vi "Filter and Data Scaling.vi"(5 "Slope":dbl[](array[numeric]), 7 "Offset":dbl[](array[numeric]), 9 "Vin":dbl[](array[numeric]), 11 "error in":errorcluster) -> (4 "Vout":dbl[](array[numeric]), 10 "ScaledOut":dbl[](array[numeric]), 15 "error out":errorcluster)   [LabVIEW 2018]
uses:
  <vilib>/ptbypt/NI_PtbyPt.lvlib
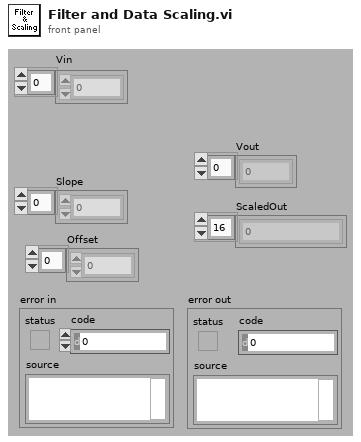
[diagram p1: front panel]
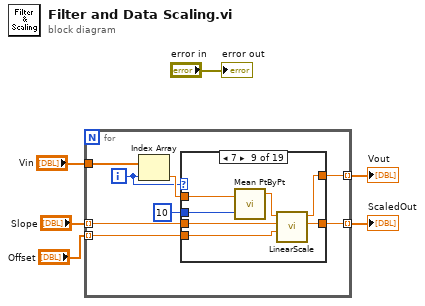
[diagram p0: block diagram]
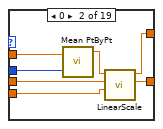
[diagram p3: hidden frame]
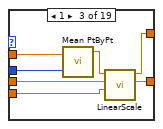
[diagram p4: hidden frame]
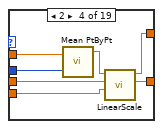
[diagram p5: hidden frame]
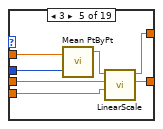
[diagram p6: hidden frame]
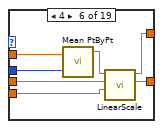
[diagram p7: hidden frame]
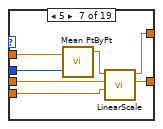
[diagram p8: hidden frame]
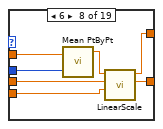
[diagram p9: hidden frame]
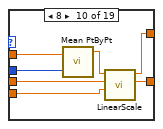
[diagram p10: hidden frame]
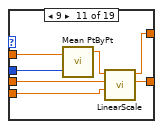
[diagram p11: hidden frame]
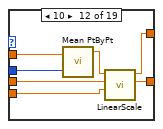
[diagram p12: hidden frame]
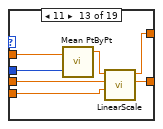
[diagram p13: hidden frame]
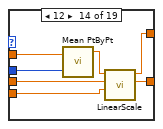
[diagram p14: hidden frame]
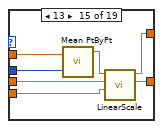
[diagram p15: hidden frame]
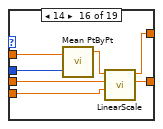
[diagram p16: hidden frame]
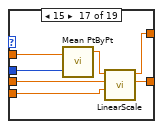
[diagram p17: hidden frame]
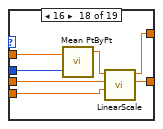
[diagram p18: hidden frame]
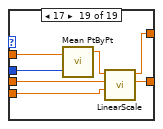
[diagram p19: hidden frame]
diagram:
  n1 = for {
    tunnel: "Slope" -> [w14] mode=indexing
    tunnel: "Offset" -> [w11] mode=indexing
    tunnel: [w12] -> w5 mode=indexing
    tunnel: [w13] -> w1 mode=indexing
    tunnel: "Vin" -> [w10]
    i -> [w8]
    n2 = Index Array(array=w10, index=w8) -> (element=w9:dbl)
    n3 = case shown="7" w8 {
      tunnel: w9 -> [_ w20 w28 w35 w42 w49 w56 w63 w70 w77 w84 w91 w98 w105 w112 w119 w126 w133 w140]
      tunnel: 10 ("String") -> [_ w15 w22 w29 w36 w43 w50 w57 w64 w71 w78 w85 w92 w99 w106 w113 w120 w127 w134]
      tunnel: w14 -> [_ w19 w26 w32 w40 w46 w53 w60 w65 w76 w82 w88 w95 w102 w110 w116 w123 w130 w137]
      tunnel: w11 -> [_ w18 w25 w33 w39 w47 w54 w61 w66 w75 w81 w89 w96 w103 w109 w117 w124 w131 w138]
      tunnel: [_ w16 w23 w31 w38 w45 w52 w59 w68 w73 w80 w87 w94 w101 w108 w115 w122 w129 w136] -> w13
      tunnel: [_ w17 w24 w30 w37 w44 w51 w58 w67 w72 w79 w86 w93 w100 w107 w114 w121 w128 w135] -> w12
      frame Default {
      }
      frame 0 {
        n4 = call <vilib>:"Mean PtByPt.vi"("x"=w20, "sample length"=w15) -> ("mean"=w21:dbl)  [unwired: 1 in, 2 out]
        n5 = call "LinearScale.vi"("Offset"=w18, "Slope"=w19, "Voltage"=w21) -> ("ScaledOut"=w17:dbl, "Vout"=w16:dbl)  [unwired: 7 in]
      }
      frame 1 {
        n6 = call <vilib>:"Mean PtByPt.vi"("x"=w28, "sample length"=w22) -> ("mean"=w27:dbl)  [unwired: 1 in, 2 out]
        n7 = call "LinearScale.vi"("Offset"=w25, "Slope"=w26, "Voltage"=w27) -> ("ScaledOut"=w24:dbl, "Vout"=w23:dbl)  [unwired: 7 in]
      }
      frame 2 {
        n8 = call <vilib>:"Mean PtByPt.vi"("x"=w35, "sample length"=w29) -> ("mean"=w34:dbl)  [unwired: 1 in, 2 out]
        n9 = call "LinearScale.vi"("Offset"=w33, "Slope"=w32, "Voltage"=w34) -> ("ScaledOut"=w30:dbl, "Vout"=w31:dbl)  [unwired: 7 in]
      }
      frame 3 {
        n10 = call <vilib>:"Mean PtByPt.vi"("x"=w42, "sample length"=w36) -> ("mean"=w41:dbl)  [unwired: 1 in, 2 out]
        n11 = call "LinearScale.vi"("Offset"=w39, "Slope"=w40, "Voltage"=w41) -> ("ScaledOut"=w37:dbl, "Vout"=w38:dbl)  [unwired: 7 in]
      }
      frame 4 {
        n12 = call <vilib>:"Mean PtByPt.vi"("x"=w49, "sample length"=w43) -> ("mean"=w48:dbl)  [unwired: 1 in, 2 out]
        n13 = call "LinearScale.vi"("Offset"=w47, "Slope"=w46, "Voltage"=w48) -> ("ScaledOut"=w44:dbl, "Vout"=w45:dbl)  [unwired: 7 in]
      }
      frame 5 {
        n14 = call <vilib>:"Mean PtByPt.vi"("x"=w56, "sample length"=w50) -> ("mean"=w55:dbl)  [unwired: 1 in, 2 out]
        n15 = call "LinearScale.vi"("Offset"=w54, "Slope"=w53, "Voltage"=w55) -> ("ScaledOut"=w51:dbl, "Vout"=w52:dbl)  [unwired: 7 in]
      }
      frame 6 {
        n16 = call <vilib>:"Mean PtByPt.vi"("x"=w63, "sample length"=w57) -> ("mean"=w62:dbl)  [unwired: 1 in, 2 out]
        n17 = call "LinearScale.vi"("Offset"=w61, "Slope"=w60, "Voltage"=w62) -> ("ScaledOut"=w58:dbl, "Vout"=w59:dbl)  [unwired: 7 in]
      }
      frame 7 {
        n18 = call <vilib>:"Mean PtByPt.vi"("x"=w70, "sample length"=w64) -> ("mean"=w69:dbl)  [unwired: 1 in, 2 out]
        n19 = call "LinearScale.vi"("Offset"=w66, "Slope"=w65, "Voltage"=w69) -> ("ScaledOut"=w67:dbl, "Vout"=w68:dbl)  [unwired: 7 in]
      }
      frame 8 {
        n20 = call <vilib>:"Mean PtByPt.vi"("x"=w77, "sample length"=w71) -> ("mean"=w74:dbl)  [unwired: 1 in, 2 out]
        n21 = call "LinearScale.vi"("Offset"=w75, "Slope"=w76, "Voltage"=w74) -> ("ScaledOut"=w72:dbl, "Vout"=w73:dbl)  [unwired: 7 in]
      }
      frame 9 {
        n22 = call <vilib>:"Mean PtByPt.vi"("x"=w84, "sample length"=w78) -> ("mean"=w83:dbl)  [unwired: 1 in, 2 out]
        n23 = call "LinearScale.vi"("Offset"=w81, "Slope"=w82, "Voltage"=w83) -> ("ScaledOut"=w79:dbl, "Vout"=w80:dbl)  [unwired: 7 in]
      }
      frame 10 {
        n24 = call <vilib>:"Mean PtByPt.vi"("x"=w91, "sample length"=w85) -> ("mean"=w90:dbl)  [unwired: 1 in, 2 out]
        n25 = call "LinearScale.vi"("Offset"=w89, "Slope"=w88, "Voltage"=w90) -> ("ScaledOut"=w86:dbl, "Vout"=w87:dbl)  [unwired: 7 in]
      }
      frame 11 {
        n26 = call <vilib>:"Mean PtByPt.vi"("x"=w98, "sample length"=w92) -> ("mean"=w97:dbl)  [unwired: 1 in, 2 out]
        n27 = call "LinearScale.vi"("Offset"=w96, "Slope"=w95, "Voltage"=w97) -> ("ScaledOut"=w93:dbl, "Vout"=w94:dbl)  [unwired: 7 in]
      }
      frame 12 {
        n28 = call <vilib>:"Mean PtByPt.vi"("x"=w105, "sample length"=w99) -> ("mean"=w104:dbl)  [unwired: 1 in, 2 out]
        n29 = call "LinearScale.vi"("Offset"=w103, "Slope"=w102, "Voltage"=w104) -> ("ScaledOut"=w100:dbl, "Vout"=w101:dbl)  [unwired: 7 in]
      }
      frame 13 {
        n30 = call <vilib>:"Mean PtByPt.vi"("x"=w112, "sample length"=w106) -> ("mean"=w111:dbl)  [unwired: 1 in, 2 out]
        n31 = call "LinearScale.vi"("Offset"=w109, "Slope"=w110, "Voltage"=w111) -> ("ScaledOut"=w107:dbl, "Vout"=w108:dbl)  [unwired: 7 in]
      }
      frame 14 {
        n32 = call <vilib>:"Mean PtByPt.vi"("x"=w119, "sample length"=w113) -> ("mean"=w118:dbl)  [unwired: 1 in, 2 out]
        n33 = call "LinearScale.vi"("Offset"=w117, "Slope"=w116, "Voltage"=w118) -> ("ScaledOut"=w114:dbl, "Vout"=w115:dbl)  [unwired: 7 in]
      }
      frame 15 {
        n34 = call <vilib>:"Mean PtByPt.vi"("x"=w126, "sample length"=w120) -> ("mean"=w125:dbl)  [unwired: 1 in, 2 out]
        n35 = call "LinearScale.vi"("Offset"=w124, "Slope"=w123, "Voltage"=w125) -> ("ScaledOut"=w121:dbl, "Vout"=w122:dbl)  [unwired: 7 in]
      }
      frame 16 {
        n36 = call <vilib>:"Mean PtByPt.vi"("x"=w133, "sample length"=w127) -> ("mean"=w132:dbl)  [unwired: 1 in, 2 out]
        n37 = call "LinearScale.vi"("Offset"=w131, "Slope"=w130, "Voltage"=w132) -> ("ScaledOut"=w128:dbl, "Vout"=w129:dbl)  [unwired: 7 in]
      }
      frame 17 {
        n38 = call <vilib>:"Mean PtByPt.vi"("x"=w140, "sample length"=w134) -> ("mean"=w139:dbl)  [unwired: 1 in, 2 out]
        n39 = call "LinearScale.vi"("Offset"=w138, "Slope"=w137, "Voltage"=w139) -> ("ScaledOut"=w135:dbl, "Vout"=w136:dbl)  [unwired: 7 in]
      }
    }
  }
  "ScaledOut" <- w5
  "Vout" <- w1
  "error out" <- "error in"
